vi "ReadBuffers.vi"(8 "error in (no error)":errorcluster, 10 "VISA resource name in":refnum<visa-resource-name>, 11 "XYGraph in":refnum<vi>) -> (0 "error out":errorcluster, 1 "Cluster":T1, 2 "Array":dbl[][](array[numeric]), 3 "VISA Refnum out":refnum<visa-resource-name>)   [LabVIEW 2020]
uses:
  Keithley 2600 Series/Keithley 2600 Series.lvlib
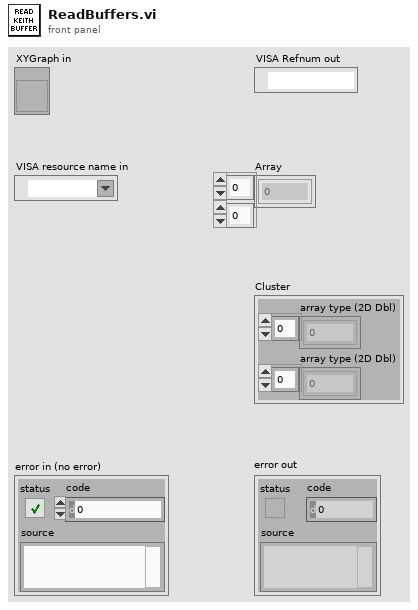
[diagram p1: front panel]
types:
  T1 = cluster{"array type (2D Dbl)":dbl[], "array type (2D Dbl)":dbl[]}
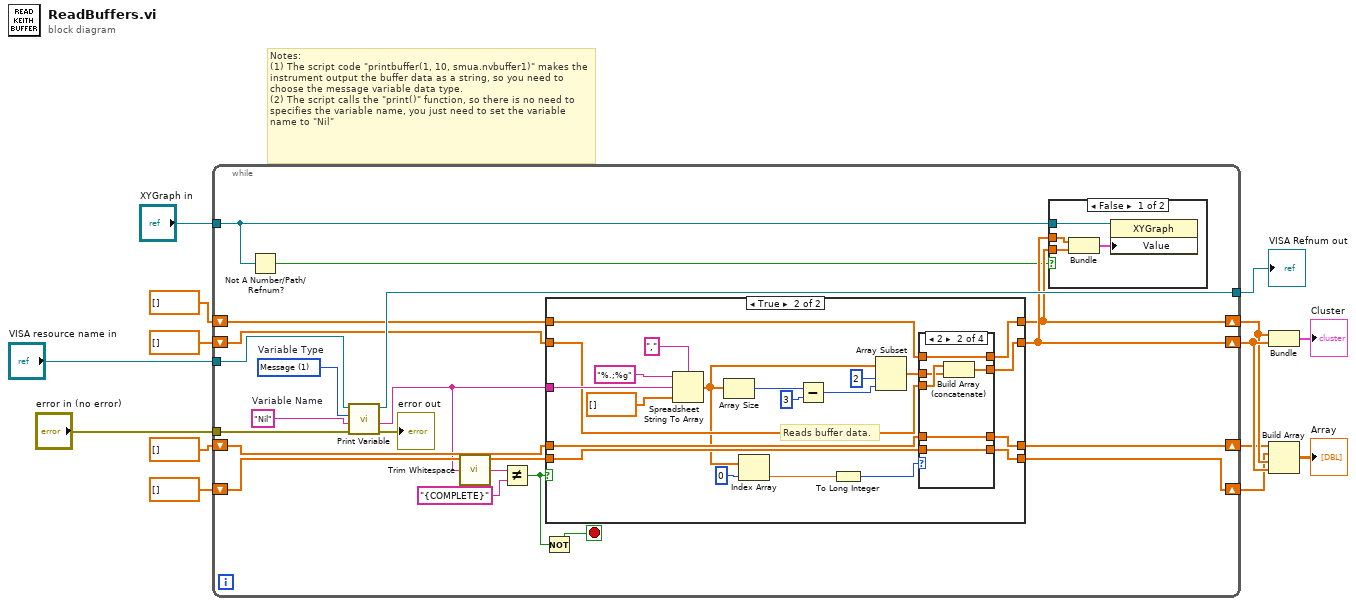
[diagram p0: block diagram]
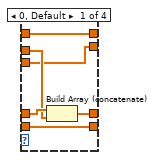
[diagram p4: hidden frame]
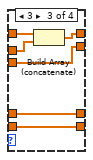
[diagram p5: hidden frame]
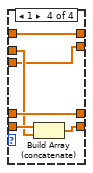
[diagram p6: hidden frame]
diagram:
  # "Notes: \n(1) The script code \"printbuffer(1, 10, smua.nvbuffer1)\" makes the instrument output the buffer data as a string, so you need to choose the message variable data type.\n(2) The script calls the \"print()\" function, so there is no need to specifies the variable name, you just need to set the variable name to \"Nil\""
  n1 = while {
    tunnel: "VISA resource name in" -> [w33]
    tunnel: "error in (no error)" -> [w32]
    tunnel: [w30] -> w3
    shift-right: [w25] -> w9
    shift-left: dbl[] [] ("array type (2D Dbl)") -> [w26]
    shift-right: [w17] -> w11
    shift-left: dbl[] [] ("array type (2D Dbl)") -> [w24]
    shift-right: [w29] -> w8
    shift-left: dbl[] [] ("array type (2D Dbl)") -> [w28]
    shift-right: [w18] -> w12
    shift-left: dbl[] [] ("array type (2D Dbl)") -> [w27]
    tunnel: "XYGraph in" -> [w16]
    stop <- w19 stop-if-true
    w35 = 1 items=["Number", "Message"]  # Variable Type
    w34 = "Nil"  # Variable Name
    n2 = Not A Number/Path/Refnum?(number/path/refnum=w16) -> (NaN/Path/Refnum?=w15:bool)
    n3 = call "Print Variable.vi"("error in (no error)"=w32, "Variable Name"=w34, "Variable Type (0: Number)"=w35, "VISA resource name"=w33) -> ("error out"=→"error out":errorcluster, "Message"=w23:string, "VISA resource name out"=w30:refnum<visa-resource-name>)  [unwired: 4 in, 1 out]
    n4 = call <vilib>:"Trim Whitespace.vi"("string"=w23) -> ("trimmed string"=w22:string)  [unwired: 1 in]
    n5 = Not Equal?(x=w22, y="{COMPLETE}") -> (x != y?=w20:bool)
    n6 = Not(x=w20) -> (.not. x?=w19:bool)
    n7 = case shown="True" w20 {
      tunnel: w23 -> [_ w61]
      tunnel: [w43 w59] -> w29
      tunnel: w28 -> [w43 w58]
      tunnel: [w41 w56] -> w18
      tunnel: w27 -> [w41 w54]
      tunnel: w26 -> [w42 w53]
      tunnel: [w42 w52] -> w25
      tunnel: w24 -> [w40 w51]
      tunnel: [w40 w50] -> w17
      frame False {
      }
      frame True {
        # "Reads buffer data."
        n8 = Spreadsheet String To Array(delimiter (Tab)=",", format string="%.;%g", spreadsheet string=w61, array type (2D Dbl)=dbl[] []) -> (array=w47:dbl[])
        n9 = Array Size(array=w47) -> (size(s)=w46:i32)
        n10 = Index Array(array=w47, index=0) -> (element=w57:dbl)
        n11 = Subtract(x=w46, y=3) -> (x-y=w44:i32)
        n12 = To Long Integer(number=w57) -> (32bit integer=w55:i32)
        n13 = Array Subset(array=w47, index=2, length=w44) -> (w49:dbl[])
        n14 = case shown="2" w55 {
          tunnel: [w68 w76 w82 w88] -> w59
          tunnel: w58 -> [w70 w76 w82 w88]
          tunnel: [w67 w71 w81 w84] -> w56
          tunnel: w49 -> [w69 w74 w78 w86]
          tunnel: w54 -> [w67 w75 w81 w84]
          tunnel: w53 -> [w66 w73 w80 w87]
          tunnel: [w66 w73 w80 w85] -> w52
          tunnel: w51 -> [w65 w72 w79 w83]
          tunnel: [w65 w72 w77 w83] -> w50
          frame 0, Default {
            n15 = Build Array (concatenate)(w70, w69) -> (w68:dbl[])
          }
          frame 2 {
            n16 = Build Array (concatenate)(w75, w74) -> (w71:dbl[])
          }
          frame 3 {
            n17 = Build Array (concatenate)(w79, w78) -> (w77:dbl[])
          }
          frame 1 {
            n18 = Build Array (concatenate)(w87, w86) -> (w85:dbl[])
          }
        }
      }
    }
    n19 = case shown="False" w15 {
      tunnel: w18 -> [w38 _]
      tunnel: w17 -> [w37 _]
      tunnel: w16 -> [w36 _]
      frame False {
        n20 = Bundle("array type (2D Dbl)"=w38, "array type (2D Dbl)"=w37) -> (w39:T1)  [unwired: 1 in]
        n21 = property class="XYGraph"(reference=w36, "Value"=w39) -> ()  [unwired: 1 in, 2 out]
      }
      frame True {
      }
    }
  }
  "VISA Refnum out" <- w3
  n22 = Bundle("array type (2D Dbl)"=w11, "array type (2D Dbl)"=w12) -> (→"Cluster":T1)  [unwired: 1 in]
  n23 = Build Array(w8, w9, w11, w12) -> (→"Array":dbl[][])
